vi "S7 Open.vi"(7 "PLC type":T1(ring), 8 "Error In":errorcluster, 9 "Slot":u8, 10 "Rack":u8, 11 "remote address":string="192.168.0.1") -> (0 "error out":errorcluster caption="Error Out", 2 "OK？":bool, 3 "TCP Out":refnum<k5>)   [LabVIEW 2020]
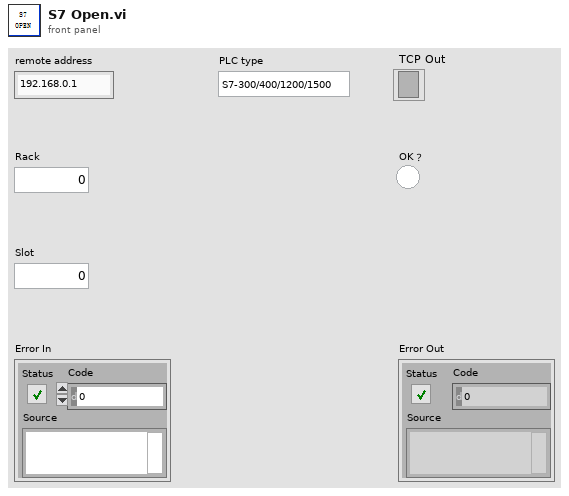
[diagram p1: front panel]
types:
  T1 = enum16{"S7-300/400/1200/1500", "S7-200", "S7-200Smart"}
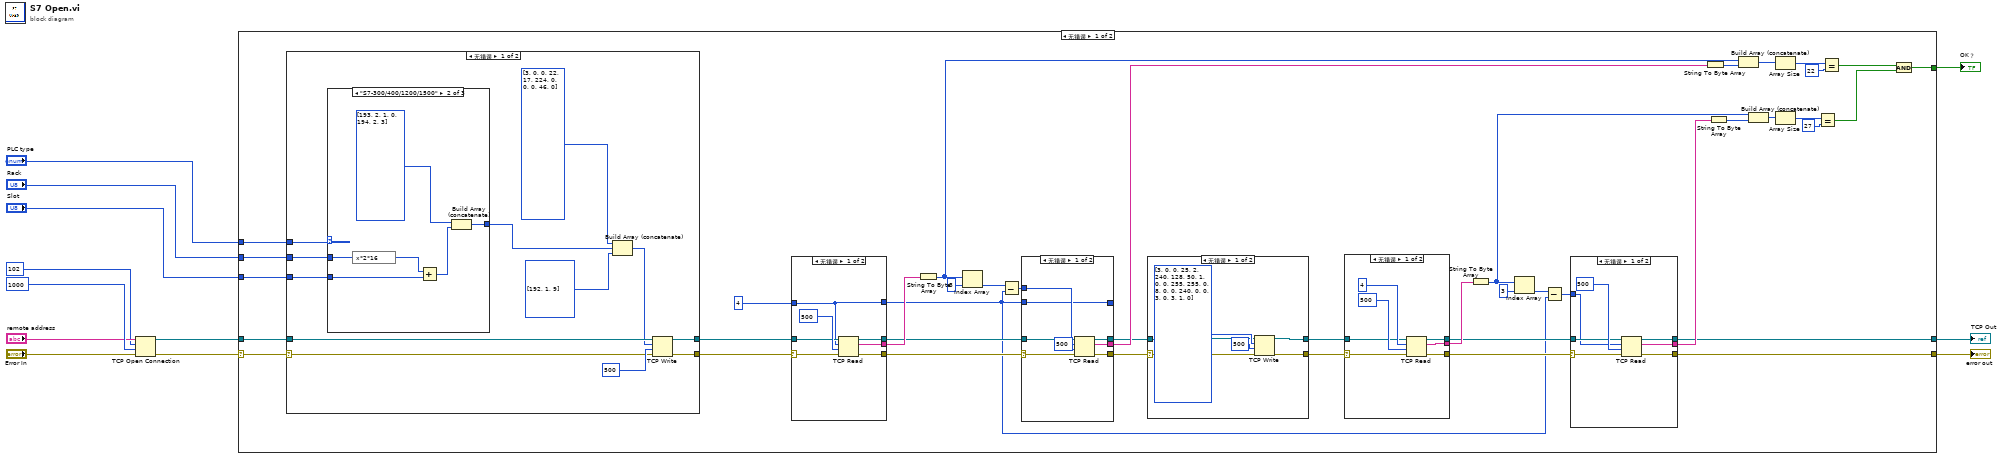
[diagram p0: block diagram]
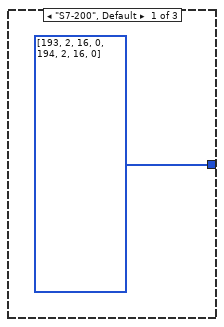
[diagram p7: hidden frame]
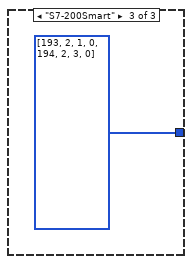
[diagram p8: hidden frame]
diagram:
  n1 = TCP Open Connection(address="remote address", remote port or service name=u16 102 ("remote port"), timeout ms (60000)=1000 ("timeout ms"), error in (no error)="Error In") -> (connection ID=w11:refnum<k5>, error out=w7:errorcluster)  [unwired: 1 out]
  n2 = case shown="无错误" w7 {
    selector: w7 -> [w23 w124]
    tunnel: [w52 w124] -> w5
    tunnel: [w47 w125] -> w12
    tunnel: w11 -> [w46 w125]
    tunnel: [w17 _] -> w4
    tunnel: "PLC type" -> [w16 _]
    tunnel: "Rack" -> [w15 _]
    tunnel: "Slot" -> [w14 _]
    frame No Error {
      n3 = case shown="无错误" w23 {
        selector: w23 -> [w105 w122]
        tunnel: [w113 w122] -> w22
        tunnel: w46 -> [w112 w123]
        tunnel: [w111 w123] -> w45
        tunnel: w16 -> [w104 _]
        tunnel: w15 -> [w103 _]
        tunnel: w14 -> [w102 _]
        frame No Error {
          n4 = case shown="\"S7-300/400/1200/1500\"" w104 {
            tunnel: [u8[] [193, 2, 16, 0, 194, 2, 16, 0] w117 u8[] [193, 2, 1, 0, 194, 2, 3, 0]] -> w110
            tunnel: w103 -> [_ w116 _]
            tunnel: w102 -> [_ w115 _]
            frame "S7-200", Default {
            }
            frame "S7-300/400/1200/1500" {
              n5 = expression code="x*2*16"(w116) -> (w120:u8)
              n6 = Add(x=w120, y=w115) -> (x+y=w118:u8)
              n7 = Build Array (concatenate)(u8[] [193, 2, 1, 0, 194, 2, 3], w118) -> (w117:u8[])
            }
            frame "S7-200Smart" {
            }
          }
          n8 = Build Array (concatenate)(u8[] [3, 0, 0, 22, 17, 224, 0, 0, 0, 46, 0] ("元素"), w110, u8[] [192, 1, 9] ("元素")) -> (w107:u8[])
          n9 = TCP Write(connection ID=w112, data in=w107, error in (no error)=w105, 9:500 ("timeout ms (25000)")) -> (connection ID out=w111:refnum<k5>, error out=w113:errorcluster)  [unwired: 1 out]
        }
        frame Error {
        }
      }
      n10 = case shown="无错误" w22 {
        selector: w22 -> [w93 w100]
        tunnel: [w97 w100] -> w21
        tunnel: [w96 _] -> w48
        tunnel: w45 -> [w95 w101]
        tunnel: [w94 w101] -> w44
        tunnel: 4 ("超时毫秒(25000)") -> [w92 w99]
        tunnel: [w92 w99] -> w13
        frame No Error {
          n11 = TCP Read(connection ID=w95, bytes to read=w92, error in (no error)=w93, 9:500 ("读取的字节")) -> (connection ID out=w94:refnum<k5>, data out=w96:string, error out=w97:errorcluster)  [unwired: 1 in]
        }
        frame Error {
        }
      }
      n12 = String To Byte Array(string=w48) -> (unsigned byte array=w39:u8[])
      n13 = Index Array(array=w39, index=3 ("索引")) -> (element=w30:u8)
      n14 = Subtract(x=w30, y=w13) -> (x-y=w29:i32)
      n15 = case shown="无错误" w21 {
        selector: w21 -> [w82 w91]
        tunnel: [w88 _] -> w53
        tunnel: [w87 w91] -> w20
        tunnel: w44 -> [w86 w90]
        tunnel: [w85 w90] -> w43
        tunnel: w29 -> [w84 _]
        tunnel: [w81 w89] -> _
        tunnel: w13 -> [w81 w89]
        frame No Error {
          n16 = TCP Read(connection ID=w86, bytes to read=w84, error in (no error)=w82, 9:500 ("timeout ms (25000)")) -> (connection ID out=w85:refnum<k5>, data out=w88:string, error out=w87:errorcluster)  [unwired: 1 in]
        }
        frame Error {
        }
      }
      n17 = case shown="无错误" w20 {
        selector: w20 -> [w75 w79]
        tunnel: w43 -> [w77 w80]
        tunnel: [w76 w80] -> w42
        tunnel: [w74 w79] -> w19
        frame No Error {
          n18 = TCP Write(connection ID=w77, data in=u8[] [3, 0, 0, 25, 2, 240, 128, 50, 1, 0, 0, 255, 255, 0, 8, 0, 0, 240, 0, 0, 3, 0, 3, 1, 0], error in (no error)=w75, 9:500 ("timeout ms (25000)")) -> (connection ID out=w76:refnum<k5>, error out=w74:errorcluster)  [unwired: 1 out]
        }
        frame Error {
        }
      }
      n19 = case shown="无错误" w19 {
        selector: w19 -> [w64 w72]
        tunnel: [w68 w72] -> w18
        tunnel: [w67 _] -> w51
        tunnel: w42 -> [w66 w71]
        tunnel: [w65 w71] -> w41
        frame No Error {
          n20 = TCP Read(connection ID=w66, bytes to read=4 ("超时毫秒(25000)"), error in (no error)=w64, 9:500 ("读取的字节")) -> (connection ID out=w65:refnum<k5>, data out=w67:string, error out=w68:errorcluster)  [unwired: 1 in]
        }
        frame Error {
        }
      }
      n21 = String To Byte Array(string=w51) -> (unsigned byte array=w37:u8[])
      n22 = Index Array(array=w37, index=3 ("索引")) -> (element=w28:u8)
      n23 = Subtract(x=w28, y=w13) -> (x-y=w26:i32)
      n24 = case shown="无错误" w18 {
        selector: w18 -> [w55 w62]
        tunnel: [w60 _] -> w54
        tunnel: [w59 w62] -> w52
        tunnel: [w58 w63] -> w47
        tunnel: w41 -> [w57 w63]
        tunnel: w26 -> [w56 _]
        frame No Error {
          n25 = TCP Read(connection ID=w57, bytes to read=w56, error in (no error)=w55, 9:500 ("读取的字节")) -> (connection ID out=w58:refnum<k5>, data out=w60:string, error out=w59:errorcluster)  [unwired: 1 in]
        }
        frame Error {
        }
      }
      n26 = String To Byte Array(string=w53) -> (unsigned byte array=w40:u8[])
      n27 = String To Byte Array(string=w54) -> (unsigned byte array=w38:u8[])
      n28 = Build Array (concatenate)(w39, w40) -> (w36:u8[])
      n29 = Build Array (concatenate)(w37, w38) -> (w32:u8[])
      n30 = Array Size(array=w36) -> (size(s)=w35:i32)
      n31 = Array Size(array=w32) -> (size(s)=w31:i32)
      n32 = Equal?(x=w31, y=27) -> (x = y?=w24:bool)
      n33 = Equal?(x=w35, y=22) -> (x = y?=w25:bool)
      n34 = And(x=w25, y=w24) -> (x .and. y?=w17:bool)
    }
    frame Error {
    }
  }
  "TCP Out" <- w12
  "error out" <- w5
  "OK？" <- w4
